vi "Eurotherm 35xx Series Temperature Control Monitoring.vi"() -> ()   [LabVIEW 2014]
doc: "This example demonstrates temperature control and monitoring.\n\nNote:\nBefore start this VI is it necessary:\n- allowed used blocks in Instrument Options (by Eurotherm iTools or by instrument front panel controls)\n- preconfigured some specific parameters this are not supported by this driver (e.g. PV-I/O Type, Linearization type, Alarm Input Values... ) by Eurotherm iTools or by instrument front panel controls\n- enter correct VISA Resource Descriptor and Device Address into front-panel controls"
uses:
  <instrlib>/Eurotherm 35xx Series/Eurotherm 35xx Series.lvlib
panel:
  in  "stop":bool
  out "Process Value - Chart":i16(graph)
  out "Process Value":i16
  in  "Setpoint Value":i16(slide) min=0 max=1300 scale=0.0..500.0
  in  "Controller Mode":u8(ring) items=["Auto", "Manual"]
  in  "Unit Address (1)":u8=1
  in  "VISA resource name":refnum<visa-resource-name>
  in  "Acknowledge All Alarms":bool
  out "ALARM !":bool
  out "Processor Utilisation in %":u8(slide) scale=0.0..100.0
  in  "Key Lock":bool
  # "(c) 2005-2010 NATIONAL INSTRUMENTS.  ALL RIGHTS RESERVED."
  # "Unlock"
  # "Lock"
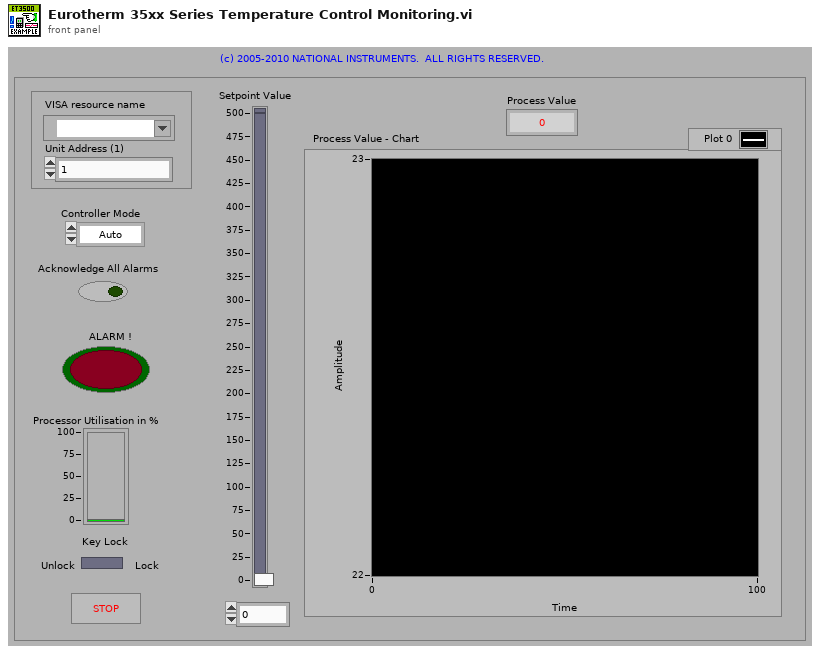
[diagram p1: front panel]
types:
  T1 = cluster{"Baud Rate (19200)":u32, "Parity (0: None)":u16, "Break Length (0)":u16}
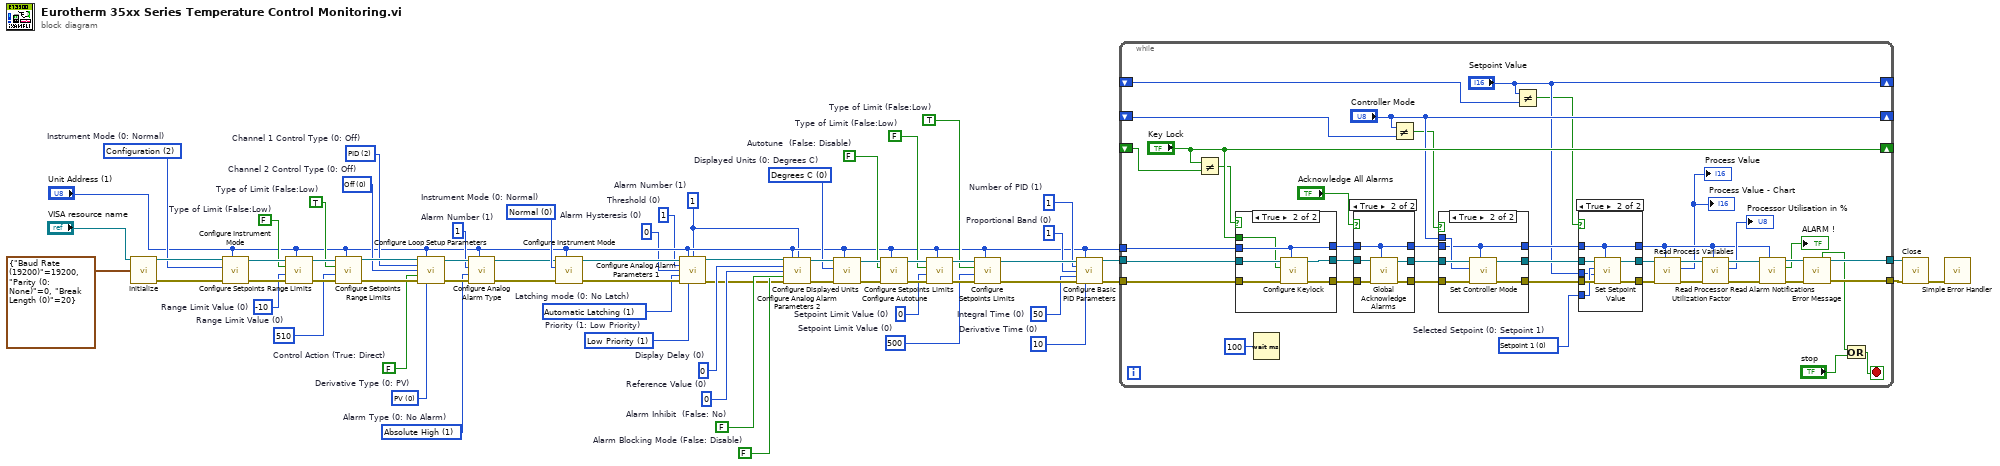
[diagram p0: block diagram]
diagram:
  w14 = 10  # Derivative Time (0)
  w15 = 50  # Integral Time (0)
  w16 = 1  # Proportional Band (0)
  w17 = u8 1  # Number of PID (1)
  w19 = i16 500  # Setpoint Limit Value (0)
  w20 = TRUE  # Type of Limit (False:Low)
  w21 = i16 0  # Setpoint Limit Value (0)
  w22 = FALSE  # Type of Limit (False:Low)
  w29 = FALSE  # Autotune  (False: Disable)
  w30 = u8 0 items=[" Degrees C", " Degrees F", " Degrees K"]  # Displayed Units (0: Degrees C)
  w37 = FALSE  # Alarm Blocking Mode (False: Disable)
  w38 = FALSE  # Alarm Inhibit  (False: No)
  w39 = 0  # Reference Value (0)
  w40 = u32 0  # Display Delay (0)
  w2 = u8 1 items=["Low Priority"=1, "Medium Priority"=2, "High Priority"=3]  # Priority (1: Low Priority)
  w3 = u16 1 items=["No Latch", "Automatic Latching", "Manual Latching", "Event Latching"]  # Latching mode (0: No Latch)
  w4 = u32 0  # Alarm Hysteresis (0)
  w5 = u32 1  # Threshold (0)
  w6 = u16 1  # Alarm Number (1)
  w41 = u8 1 items=["No Alarm", "Absolute High", "Absolute Low", "Deviation High", "Deviation Low", "Deviation Band", "Rising Rate of Change Alarm", "Falling Rate of Change Alarm"]  # Alarm Type (0: No Alarm)
  w42 = u16 1  # Alarm Number (1)
  w47 = u8 0 items=["Normal", "StandBy", "Configuration"]  # Instrument Mode (0: Normal)
  w48 = u8 0 items=["PV", "Error"]  # Derivative Type (0: PV)
  w49 = FALSE  # Control Action (True: Direct)
  w50 = u8 0 items=["Off", "On/Off", "PID", "VPU", "VPB"]  # Channel 2 Control Type (0: Off)
  w51 = u8 2 items=["Off", "On/Off", "PID", "VPU", "VPB"]  # Channel 1 Control Type (0: Off)
  w54 = TRUE  # Type of Limit (False:Low)
  w55 = 510  # Range Limit Value (0)
  w58 = -10  # Range Limit Value (0)
  w59 = FALSE  # Type of Limit (False:Low)
  w62 = u8 2 items=["Normal", "StandBy", "Configuration"]  # Instrument Mode (0: Normal)
  n1 = call <instrlib>:"Initialize.vi"("VISA resource name"="VISA resource name", "Serial Configuration"=T1 {"Baud Rate (19200)"=19200, "Parity (0: None)"=0, "Break Length (0)"=20}) -> ("VISA resource name out"=w63:refnum<visa-resource-name>, "error out"=w12:errorcluster)  [unwired: 12 in]
  n2 = call <instrlib>:"Configure Instrument Mode.vi"("Unit Address (1)"="Unit Address (1)", "error in (no error)"=w12, "Instrument Mode (0: Normal)"=w62, "VISA resource name"=w63) -> ("error out"=w60:errorcluster, "VISA resource name out"=w61:refnum<visa-resource-name>)  [unwired: 6 in]
  n3 = call <instrlib>:"Configure Setpoints Range Limits.vi"("Unit Address (1)"="Unit Address (1)", "error in (no error)"=w60, "Range Limit Value (0)"=w58, "Limit Type (False)"=w59, "VISA resource name"=w61) -> ("error out"=w57:errorcluster, "VISA resource name out"=w56:refnum<visa-resource-name>)  [unwired: 5 in]
  n4 = call <instrlib>:"Configure Setpoints Range Limits.vi"("Unit Address (1)"="Unit Address (1)", "error in (no error)"=w57, "Range Limit Value (0)"=w55, "Limit Type (False)"=w54, "VISA resource name"=w56) -> ("error out"=w52:errorcluster, "VISA resource name out"=w53:refnum<visa-resource-name>)  [unwired: 5 in]
  n5 = call <instrlib>:"Configure Loop Setup Parameters.vi"("VISA resource name"=w53, "Unit Address (1)"="Unit Address (1)", "Channel 1 Control Type (0: Off)"=w51, "Channel 2 Control Type (0: Off)"=w50, "Control Action (True: Direct)"=w49, "error in (no error)"=w52, "Derivative Type (0: PV)"=w48) -> ("VISA resource name out"=w46:refnum<visa-resource-name>, "error out"=w45:errorcluster)  [unwired: 7 in]
  n6 = call <instrlib>:"Configure Analog Alarm Type.vi"("Unit Address (1)"="Unit Address (1)", "error in (no error)"=w45, "Alarm Type (0: No Alarm)"=w41, "Alarm Number (1)"=w42, "VISA resource name"=w46) -> ("error out"=w43:errorcluster, "VISA resource name out"=w44:refnum<visa-resource-name>)  [unwired: 5 in]
  n7 = call <instrlib>:"Configure Instrument Mode.vi"("Unit Address (1)"="Unit Address (1)", "error in (no error)"=w43, "Instrument Mode (0: Normal)"=w47, "VISA resource name"=w44) -> ("error out"=w8:errorcluster, "VISA resource name out"=w11:refnum<visa-resource-name>)  [unwired: 6 in]
  n8 = call <instrlib>:"Configure Analog Alarm Parameters 1.vi"("VISA resource name"=w11, "Unit Address (1)"="Unit Address (1)", "Alarm Number (1)"=w6, "Threshold (0)"=w5, "Alarm Hysteresis (0)"=w4, "Latching Mode (0: No Latch)"=w3, "error in (no error)"=w8, "Priority (1: Low Priority)"=w2) -> ("VISA resource name out"=w10:refnum<visa-resource-name>, "error out"=w9:errorcluster)  [unwired: 6 in]
  n9 = call <instrlib>:"Configure Analog Alarm Parameters 2.vi"("VISA resource name"=w10, "Unit Address (1)"="Unit Address (1)", "Alarm Number (1)"=w6, "Display Delay (0)"=w40, "Reference Value (0)"=w39, "Alarm Inhibit  (False:Disable)"=w38, "error in (no error)"=w9, "Alarm Blocking Mode (False: Disable)"=w37) -> ("VISA resource name out"=w36:refnum<visa-resource-name>, "error out"=w35:errorcluster)  [unwired: 6 in]
  n10 = call <instrlib>:"Configure Displayed Units.vi"("Unit Address (1)"="Unit Address (1)", "error in (no error)"=w35, "Displayed Units (0: Degrees C)"=w30, "VISA resource name"=w36) -> ("error out"=w33:errorcluster, "VISA resource name out"=w34:refnum<visa-resource-name>)  [unwired: 6 in]
  n11 = call <instrlib>:"Configure Autotune.vi"("Unit Address (1)"="Unit Address (1)", "error in (no error)"=w33, "Autotune  (False: Disable)"=w29, "VISA resource name"=w34) -> ("error out"=w27:errorcluster, "VISA resource name out"=w28:refnum<visa-resource-name>)  [unwired: 6 in]
  n12 = call <instrlib>:"Configure Setpoints Limits.vi"("Unit Address (1)"="Unit Address (1)", "error in (no error)"=w27, "Setpoint Limit Value (0)"=w21, "Limit Type (False)"=w22, "VISA resource name"=w28) -> ("error out"=w31:errorcluster, "VISA resource name out"=w32:refnum<visa-resource-name>)  [unwired: 5 in]
  n13 = call <instrlib>:"Configure Setpoints Limits.vi"("Unit Address (1)"="Unit Address (1)", "error in (no error)"=w31, "Setpoint Limit Value (0)"=w19, "Limit Type (False)"=w20, "VISA resource name"=w32) -> ("error out"=w23:errorcluster, "VISA resource name out"=w26:refnum<visa-resource-name>)  [unwired: 5 in]
  n14 = call <instrlib>:"Configure Basic PID Parameters.vi"("VISA resource name"=w26, "Unit Address (1)"="Unit Address (1)", "PID Number  (1)"=w17, "Proportional Band (0)"=w16, "Integral Time (0)"=w15, "error in (no error)"=w23, "Derivative Time (0)"=w14) -> ("VISA resource name out"=w25:refnum<visa-resource-name>, "error out"=w24:errorcluster)  [unwired: 7 in]
  n15 = while {
    tunnel: w25 -> [w67]
    tunnel: w24 -> [w66]
    tunnel: "Unit Address (1)" -> [w68]
    tunnel: [w92] -> w13
    tunnel: [w91] -> w18
    shift-right: ["Key Lock"] -> _
    shift-left: _ -> [w78]
    shift-right: ["Controller Mode"] -> _
    shift-left: _ -> [w74]
    shift-right: ["Setpoint Value"] -> _
    shift-left: _ -> [w72]
    stop <- w82 stop-if-true
    w86 = u8 0 items=["Setpoint 1", "Setpoint 2", "Alternate Setpoint", "Target Setpoint"]  # Selected Setpoint (0: Setpoint 1)
    n16 = Not Equal?(x="Key Lock", y=w78) -> (x != y?=w76:bool)
    n17 = case shown="True" w76 {
      tunnel: w67 -> [w135 w142]
      tunnel: w66 -> [w134 w141]
      tunnel: [w135 w140] -> w100
      tunnel: [w134 w139] -> w99
      tunnel: w68 -> [w136 w138]
      tunnel: [w136 w138] -> w88
      tunnel: "Key Lock" -> [_ w137]
      frame False {
      }
      frame True {
        n18 = call <instrlib>:"Configure Keylock.vi"("Unit Address (1)"=w138, "error in (no error)"=w141, "Enable Keylock (False: Unlock)"=w137, "VISA resource name"=w142) -> ("error out"=w139:errorcluster, "VISA resource name out"=w140:refnum<visa-resource-name>)  [unwired: 6 in]
      }
    }
    n19 = Wait (ms)(milliseconds to wait=u32 100) -> ()  [unwired: 1 out]
    n20 = case shown="True" "Acknowledge All Alarms" {
      tunnel: w100 -> [w127 w133]
      tunnel: w99 -> [w126 w132]
      tunnel: [w127 w131] -> w94
      tunnel: [w126 w130] -> w93
      tunnel: w88 -> [w128 w129]
      tunnel: [w128 w129] -> w87
      frame False {
      }
      frame True {
        n21 = call <instrlib>:"Global  Acknowledge Alarms.vi"("Unit Address (1)"=w129, "error in (no error)"=w132, "VISA resource name"=w133) -> ("error out"=w130:errorcluster, "VISA resource name out"=w131:refnum<visa-resource-name>)  [unwired: 7 in]
      }
    }
    n22 = Not Equal?(x="Controller Mode", y=w74) -> (x != y?=w73:bool)
    n23 = case shown="True" w73 {
      tunnel: [w117 w125] -> w98
      tunnel: [w118 w124] -> w95
      tunnel: w94 -> [w118 w123]
      tunnel: w93 -> [w117 w122]
      tunnel: w87 -> [w119 w120]
      tunnel: "Controller Mode" -> [_ w121]
      tunnel: [w119 w120] -> w85
      frame False {
      }
      frame True {
        n24 = call <instrlib>:"Set Controller Mode.vi"("Unit Address (1)"=w120, "error in (no error)"=w122, "Controller Mode (0: Auto)"=w121, "VISA resource name"=w123) -> ("error out"=w125:errorcluster, "VISA resource name out"=w124:refnum<visa-resource-name>)  [unwired: 6 in]
      }
    }
    n25 = Not Equal?(x="Setpoint Value", y=w72) -> (x != y?=w70:bool)
    n26 = case shown="True" w70 {
      tunnel: w98 -> [w107 w116]
      tunnel: [w107 w115] -> w97
      tunnel: [w108 w114] -> w96
      tunnel: w95 -> [w108 w113]
      tunnel: w86 -> [_ w112]
      tunnel: w85 -> [w109 w111]
      tunnel: [w109 w111] -> w84
      tunnel: "Setpoint Value" -> [_ w110]
      frame False {
      }
      frame True {
        n27 = call <instrlib>:"Set Setpoint Value.vi"("Unit Address (1)"=w111, "error in (no error)"=w116, "Setpoint Value (0)"=w110, "Selected Setpoint (0: Setpoint 1)"=w112, "VISA resource name"=w113) -> ("error out"=w115:errorcluster, "VISA resource name out"=w114:refnum<visa-resource-name>)  [unwired: 5 in]
      }
    }
    n28 = call <instrlib>:"Read Process Variables.vi"("Unit Address (1)"=w84, "error in (no error)"=w97, "VISA resource name"=w96) -> ("error out"=w105:errorcluster, "Process Value"=→"Process Value" →"Process Value - Chart":i16, "VISA resource name out"=w106:refnum<visa-resource-name>)  [unwired: 5 in, 1 out]
    n29 = call <instrlib>:"Read Processor Utilization Factor.vi"("Unit Address (1)"=w84, "error in (no error)"=w105, "VISA resource name"=w106) -> ("error out"=w103:errorcluster, "Processor Utilization in %"=→"Processor Utilisation in %":u8, "VISA resource name out"=w104:refnum<visa-resource-name>)  [unwired: 6 in]
    n30 = call <instrlib>:"Read Alarm Notifications.vi"("Unit Address (1)"=w84, "error in (no error)"=w103, "VISA resource name"=w104) -> ("error out"=w101:errorcluster, "New Alarm"=→"ALARM !":bool, "VISA resource name out"=w102:refnum<visa-resource-name>)  [unwired: 5 in, 1 out]
    n31 = call <instrlib>:"Error Message.vi"("VISA resource name"=w102, "error in (no error)"=w101) -> ("Status"=w80:bool, "VISA resource name out"=w92:refnum<visa-resource-name>, "error out"=w91:errorcluster)  [unwired: 9 in, 2 out]
    n32 = Or(x=w80, y="stop") -> (x .or. y?=w82:bool)
  }
  n33 = call <instrlib>:"Close.vi"("VISA resource name"=w13, "error in (no error)"=w18) -> ("error out"=w1:errorcluster)  [unwired: 13 in]
  n34 = call <vilib>:"Simple Error Handler.vi"("error in (no error)"=w1) -> ()  [unwired: 4 in, 5 out]
